vi "W2Naturalnos.vi"() -> ()   [LabVIEW 2023]
panel:
  out "Numeric":i32
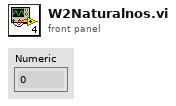
[diagram p1: front panel]
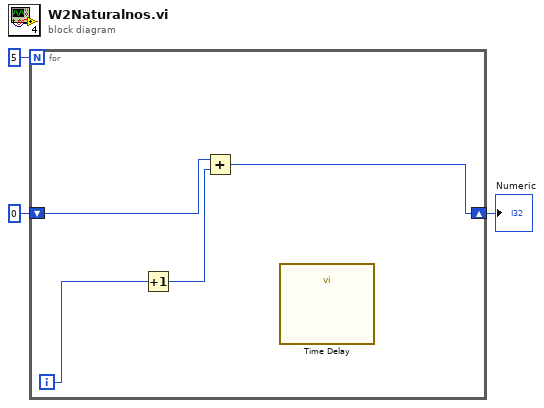
[diagram p0: block diagram]
diagram:
  n1 = for {
    N: 5 -> [_]
    shift-right: [w7] -> w1
    shift-left: 0 -> [w4]
    i -> [w6]
    n2 = Increment(x=w6) -> (x+1=w5:i32)
    n3 = Add(x=w4, y=w5) -> (x+y=w7:i32)
    n4 = call "Time Delay"() -> ()  [unwired: 11 in, 1 out]
  }
  "Numeric" <- w1
